vi "Curtin_FindBands.vi"(0 "CrsrList":T3, 1 "Labels":string[](array[string]), 2 "Excel?":bool, 3 "Magnitude":T2(graph)) -> (4 "Raw Data":T1, 5 "Cursor Data":string[][](table), 6 "Filter":T2(graph), 7 "Centroids":T2(graph))   [LabVIEW 2022 SP3]
uses:
  <vilib>/Utility/miscctls.llb/LVCursorListTypeDef.ctl
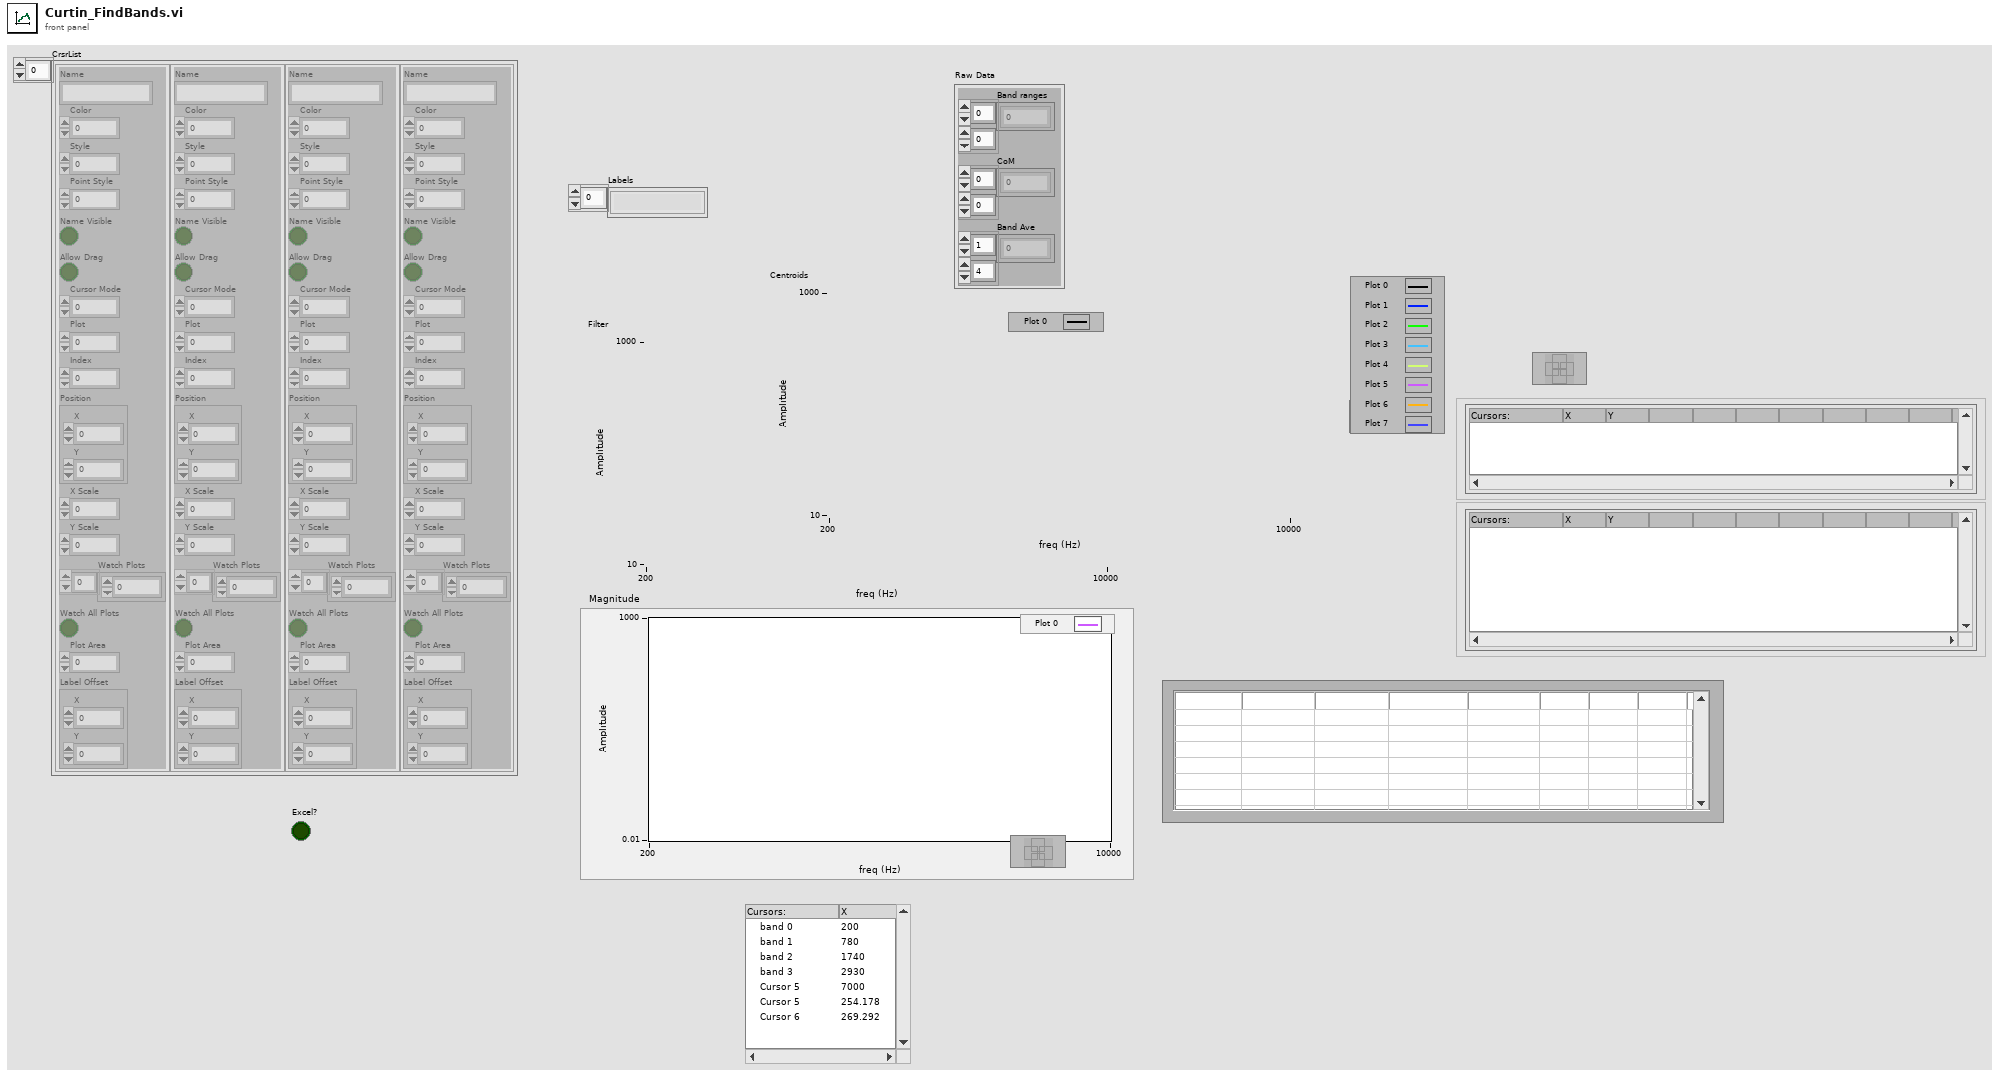
[diagram p1: front panel]
types:
  T1 = cluster{"Band ranges":dbl[][], "CoM":dbl[][], "Band Ave":dbl[][]}
  T2 = cluster{dbl, "df":dbl, "Power Spectrum (V^2 rms)":dbl[]}[]
  T3 = typedef "LVCursorListTypeDef.ctl" = cluster{"Name":string, "Color":u32, "Style":u8, "Point Style":u8, "Name Visible":bool, "Allow Drag":bool, "Cursor Mode":u32, "Plot":i32, "Index":i32, "Position":cluster{"X":dbl, "Y":dbl}, "X Scale":u32, "Y Scale":u32, "Watch Plots":i32[], "Watch All Plots":bool, "Plot Area":i32, "Label Offset":cluster{"X":dbl, "Y":dbl}}[]
  T4 = cluster{dbl, "df":dbl, "Power Spectrum (V^2 rms)":dbl[]}
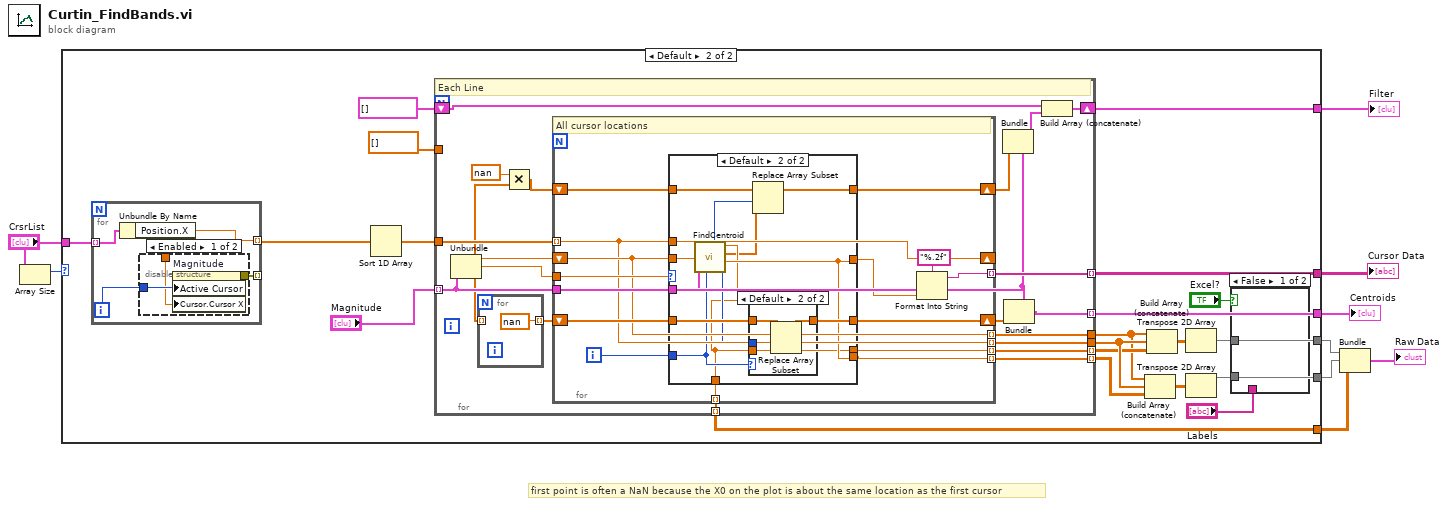
[diagram p0: block diagram]
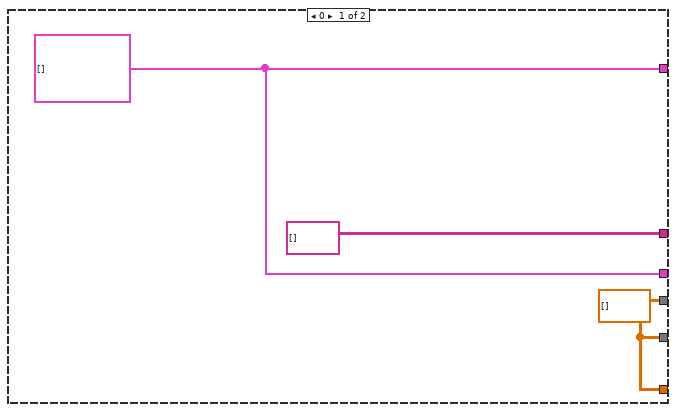
[diagram p2: hidden frame]
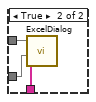
[diagram p3: hidden frame]
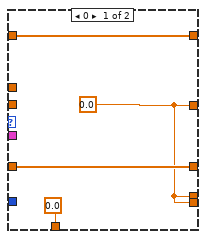
[diagram p4: hidden frame]
diagram:
  # "first point is often a NaN because the X0 on the plot is about the same location as the first cursor"
  n1 = Array Size(array="CrsrList") -> (size(s)=w7:i32)
  n2 = case shown="Default" w7 {
    tunnel: "CrsrList" -> [_ w31]
    tunnel: [w11 w30] -> w9
    tunnel: [string[][] [] w29] -> w6
    tunnel: [w11 w26] -> w5
    tunnel: [w10 w17] -> w3
    tunnel: [w10 w16] -> w4
    tunnel: [w10 w15] -> w1
    frame 0 {
      w10 = dbl[][] []
      w11 = T2 []
    }
    frame Default {
      n3 = for {
        tunnel: w31 -> [w97] mode=indexing
        tunnel: [w95] -> _ mode=indexing
        tunnel: [w94] -> w14 mode=indexing
        i -> [w96]
        n4 = Unbundle By Name(w97) -> ("Position.X"=w94:dbl)
        n5 = disable-structure shown="Enabled" {
          disable-tunnel: w96 -> [w100 _]
          disable-tunnel: [w99 _] -> w95
          disable-tunnel: w94 -> [w98 _]
          frame Enabled {
            n6 = property on="Magnitude" class="WFGraph (strict)"("Active Cursor"=w100, "Cursor.Cursor X"=w98) -> (error out=w99:errorcluster)  [unwired: 2 in, 1 out]
          }
          frame Disabled {
          }
        }
      }
      n7 = Sort 1D Array(array=w14) -> (sorted array=w13:dbl[])
      n8 = for {
        tunnel: "Magnitude" -> [w46] mode=indexing
        tunnel: dbl[] [] -> [_]
        shift-right: [w54] -> w30
        shift-left: T2 [] -> [w52]
        tunnel: [w51] -> w29 mode=indexing
        tunnel: [w45] -> w26 mode=indexing
        tunnel: [w44] -> w20
        tunnel: [w43] -> w24
        tunnel: [w42] -> w23 mode=indexing
        tunnel: [w41] -> w22 mode=indexing
        tunnel: [w40] -> w15 mode=indexing
        tunnel: w13 -> [w39]
        # "Each Line"
        n9 = Unbundle(w46) -> (w49:dbl, "df"=w50:dbl, "Power Spectrum (V^2 rms)"=w37:dbl[])
        n10 = for {
          tunnel: w37 -> [_] mode=indexing
          tunnel: [nan] -> w48 mode=indexing
        }
        n11 = Multiply(x=nan, y=w37) -> (x*y=w36:dbl[])
        n12 = for {
          shift-right: [w60] -> _
          shift-left: w49 -> [w64]
          shift-right: [w58] -> w55
          shift-left: w36 -> [w59]
          tunnel: [w70] -> w51 mode=indexing
          tunnel: w50 -> [w69]
          tunnel: w46 -> [w68]
          shift-right: [w65] -> w47
          shift-left: w48 -> [w66]
          tunnel: [w64] -> w44 mode=indexing
          tunnel: [w60] -> w43 mode=indexing
          tunnel: [w63] -> w42 mode=indexing
          tunnel: [w57] -> w41 mode=indexing
          tunnel: [w61] -> w40 mode=indexing
          tunnel: w39 -> [w60] mode=indexing
          i -> [w62]
          # "All cursor locations"
          n13 = case shown="Default" w69 {
            tunnel: w64 -> [_ w87]
            tunnel: w68 -> [_ w86]
            tunnel: w60 -> [_ w88]
            tunnel: [w74 w82] -> w67
            tunnel: w66 -> [w75 w85]
            tunnel: [w75 w84] -> w65
            tunnel: [w74 w80] -> w63
            tunnel: [w74 w82] -> w57
            tunnel: w62 -> [_ w81]
            tunnel: [0.0 ("mean") w80] -> w61
            tunnel: w59 -> [w72 w79]
            tunnel: [w72 w76] -> w58
            frame 0 {
              w74 = 0.0 ("mean")
            }
            frame Default {
              n14 = call "FindCentroid.vi"("i"=w81, "Plot"=w86, "Last PosX"=w87, "New PosX"=w88) -> ("nearest point"=w83:i32, "f Centroid"=w82:dbl, "Filter line"=w77:dbl[], "mean"=w80:dbl, "start"=w78:i32)  [unwired: 3 in]
              n15 = case shown="Default" w81 {
                tunnel: w85 -> [w89 w93]
                tunnel: [w89 w92] -> w84
                tunnel: w83 -> [_ w91]
                tunnel: w80 -> [_ w90]
                frame 0 {
                }
                frame Default {
                  n16 = Replace Array Subset(array=w93, new element=w90, index=w91) -> (w92:dbl[])
                }
              }
              n17 = Replace Array Subset(array=w79, new element=w77, index=w78) -> (w76:dbl[])
            }
          }
          n18 = Format Into String(format string="%.2f", w67) -> (resulting string=w70:string)  [unwired: 2 in, 1 out]
        }
        n19 = Bundle(cluster=w46, "Power Spectrum (V^2 rms)"=w55) -> (w53:T4)  [unwired: 2 in]
        n20 = Bundle(cluster=w46, "Power Spectrum (V^2 rms)"=w47) -> (w45:T4)  [unwired: 2 in]
        n21 = Build Array (concatenate)(w52, w53) -> (w54:T2)
      }
      n22 = Build Array (concatenate)(w20, w24, w22) -> (w21:dbl[][])
      n23 = Build Array (concatenate)(w20, w24, w23) -> (w25:dbl[][])
      n24 = Transpose 2D Array(2D array=w25) -> (transposed array=w16:dbl[][])
      n25 = Transpose 2D Array(2D array=w21) -> (transposed array=w17:dbl[][])
      n26 = case shown="False" "Excel?" {
        tunnel: w16 -> [_ w35]
        tunnel: w17 -> [_ w34]
        tunnel: "Labels" -> [_ w33]
        frame False {
        }
        frame True {
          n27 = call "ExcelDialog.vi"("Labels"=w33, "Center of Masses"=w34, "Band Average"=w35) -> ()  [unwired: 9 in]
        }
      }
    }
  }
  "Filter" <- w9
  "Cursor Data" <- w6
  "Centroids" <- w5
  n28 = Bundle(w4, w3, w1) -> (→"Raw Data":cluster{dbl[][], dbl[][], dbl[][]})  [unwired: 1 in]
